vi "CleanUp.vi"(8 "error in (no error)":errorcluster, 11 "Prueba08 in":refnum<class "Prueba31.lvclass">) -> (0 "error out":errorcluster, 3 "Prueba08 out":refnum<class "Prueba31.lvclass">)   [LabVIEW 2019, in "Prueba31.lvclass"]
uses:
  Prueba31.lvclass
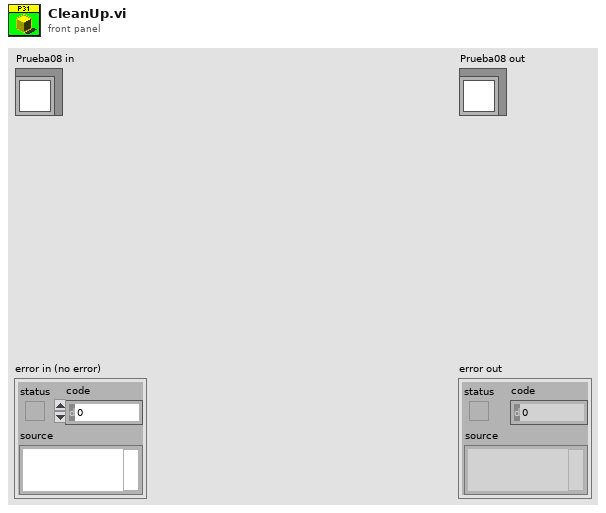
[diagram p1: front panel]
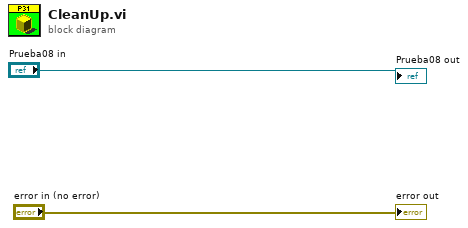
[diagram p0: block diagram]
diagram:
  "error out" <- "error in (no error)"
  "Prueba08 out" <- "Prueba08 in"
